vi "Close Connection to Shared Variables.vi"(8 "Error In":errorcluster, 11 "Page Configurations In":T2(array[cluster])) -> (0 "Error Out":errorcluster, 3 "Page Configurations Out":T2(array[cluster]))   [LabVIEW 2017, in "DTacq Plot Display Library.lvlib"]
doc: "Opens a read-only connection to every shared variable which is a part of this configuration.\n\nA connection to a shared variable must be open, before attempting to read data from it."
uses:
  DTacq Plot Display Library.lvlib
  Typedefs/Plot Channel Configruation--Cluster.ctl
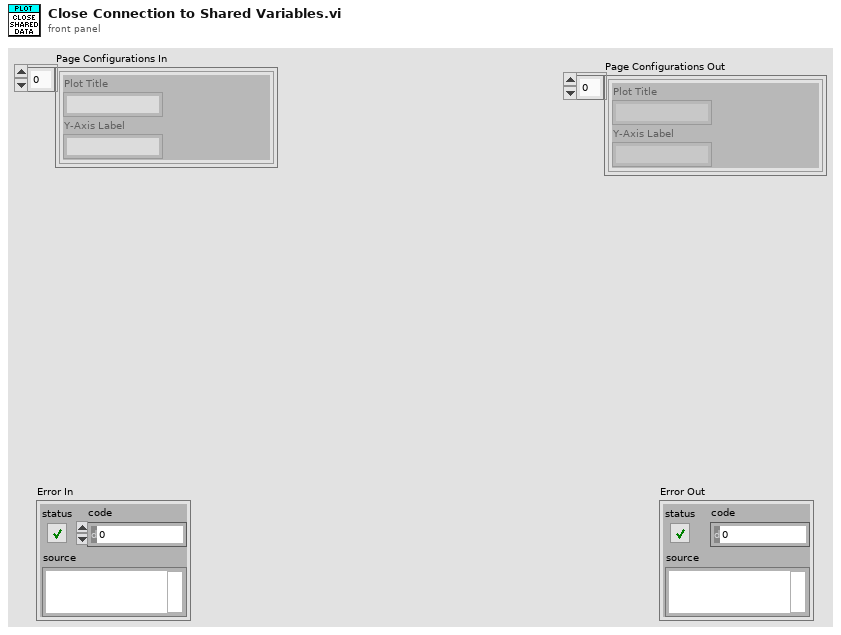
[diagram p1: front panel]
types:
  T1 = typedef "DTacq Plot Display Library.lvlib/Plot Channel Configruation--Cluster.ctl" = cluster{"Shared Variable Reference":refnum<k21>, "Full Variable Name":string, "URL":string, "Descriptive Name":string, "Data Type":variant, "Colour":u32}
  T2 = cluster{"Plot Title":string, "Y-Axis Label":string, "X-Axis Label":string, "Plot Channel Configurations":T1[]}[]
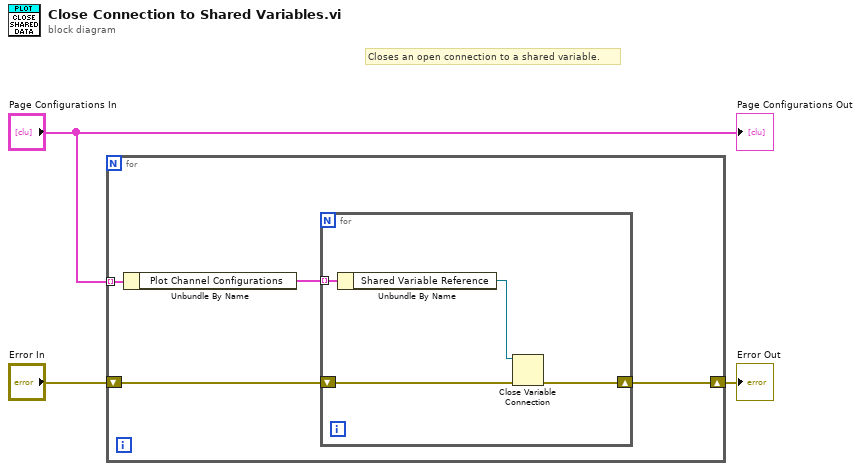
[diagram p0: block diagram]
diagram:
  # "Closes an open connection to a shared variable."
  n1 = for {
    tunnel: "Page Configurations In" -> [w4] mode=indexing
    shift-right: [w5] -> w2
    shift-left: "Error In" -> [w6]
    n2 = Unbundle By Name(w4) -> ("Plot Channel Configurations"=w7:T1[])
    n3 = for {
      tunnel: w7 -> [w11] mode=indexing
      shift-right: [w8] -> w5
      shift-left: w6 -> [w9]
      n4 = Unbundle By Name(w11) -> ("Shared Variable Reference"=w10:refnum<k21>)
      n5 = Close Variable Connection(8:w9, 11:w10) -> (0:w8:errorcluster)
    }
  }
  "Error Out" <- w2
  "Page Configurations Out" <- "Page Configurations In"
